vi "Write--home.vi"(8 "error in (no error)":errorcluster, 9 "Home direction (M2)":T1=1 items=["", "Forward", "Backward"], 10 "Home direction (M1)":T1=1 items=["", "Forward", "Backward"], 11 "VISA resource name":refnum<visa-resource-name>) -> (0 "error out":errorcluster, 1 "Comando":T2={"Action"=1, "Direction motor 1"=1, "Direction motor 2"=1, "Steps motor 1"=200, "Steps motor 2"=200, "Step style motor 1"=1, "Step style motor 2"=1} {"Step style motor 2" items=["", "Single", "Double", "Interleave", "Microstep"]; "Step style motor 1" items=["", "Single", "Double", "Interleave", "Microstep"]; "Direction motor 2" items=["", "Forward", "Backward"]; "Direction motor 1" items=["", "Forward", "Backward"]; "Action" items=["", "Initialize", "Move"]}, 2 "Comando(string)":string, 3 "VISA resource name out":refnum<visa-resource-name>)   [LabVIEW 2020, in "Control de MaP.lvlib"]
doc: "convierte la selección de comando a cadena y lo envía al puerto seleccionado"
uses:
  Control de MaP.lvlib
  Controls/Move motor parameters--cluster.ctl
  Controls/Motor direction.ctl
  Controls/Step style.ctl
  Arduino-Adafruit stepper/Arduino-Adafruit stepper.lvlib
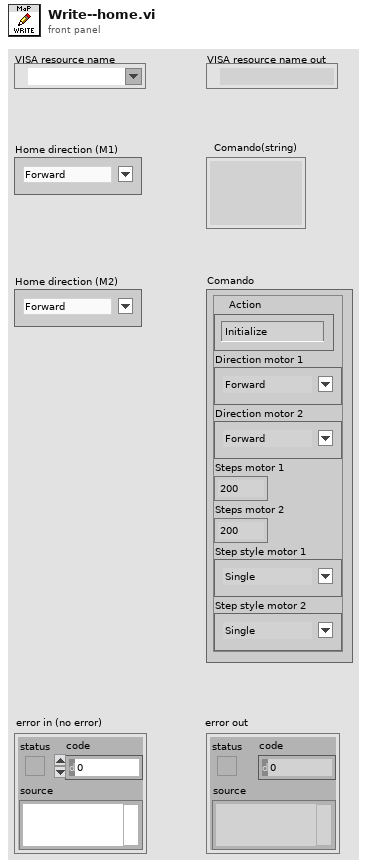
[diagram p1: front panel]
types:
  T1 = typedef "Arduino-Adafruit stepper.lvlib/Motor direction.ctl" = u8
  T2 = typedef "Arduino-Adafruit stepper.lvlib/Move motor parameters--cluster.ctl" = cluster{"Action":u8, "Direction motor 1":T1, "Direction motor 2":T1, "Steps motor 1":u16, "Steps motor 2":u16, "Step style motor 1":T3, "Step style motor 2":T3}
  T3 = typedef "Arduino-Adafruit stepper.lvlib/Step style.ctl" = u8
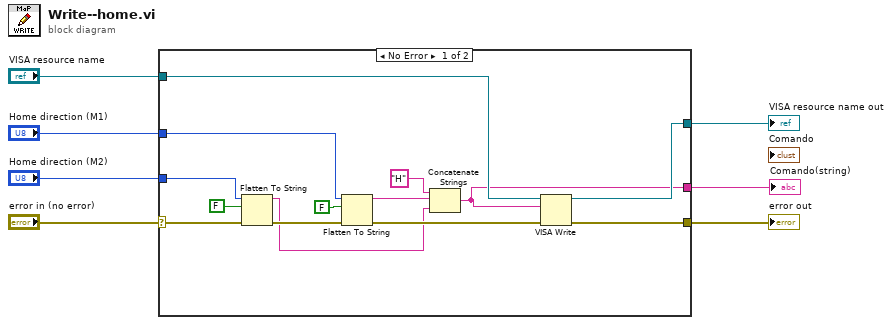
[diagram p0: block diagram]
diagram:
  n1 = case shown="No Error" "error in (no error)" {
    selector: "error in (no error)" -> [w11 w23]
    tunnel: "VISA resource name" -> [w14 w22]
    tunnel: [w21 w22] -> w6
    tunnel: [w20 w23] -> w4
    tunnel: "Home direction (M1)" -> [w17 _]
    tunnel: [w13 _] -> w2
    tunnel: "Home direction (M2)" -> [w9 _]
    frame No Error {
      n2 = Flatten To String(anything=w9, prepend array or string size? (T)=FALSE, error in (no error)=w11) -> (data string=w8:string, error out=w10:errorcluster)  [unwired: 1 in, 1 out]
      n3 = Flatten To String(anything=w17, prepend array or string size? (T)=FALSE, error in (no error)=w10) -> (data string=w16:string, error out=w18:errorcluster)  [unwired: 1 in, 1 out]
      n4 = Concatenate Strings("H", w16, w8) -> (w13:string)
      n5 = VISA Write(VISA resource name=w14, write buffer=w13, error in (no error)=w18) -> (VISA resource name out=w21:refnum<visa-resource-name>, error out=w20:errorcluster)  [unwired: 1 out]
    }
    frame Error {
    }
  }
  "VISA resource name out" <- w6
  "error out" <- w4
  "Comando(string)" <- w2
